vi "Destroy.vi"(0 "reference in":refnum<class "MessageAMC.lvclass">, 5 "error in (no error)":errorcluster) -> (14 "reference out":refnum<class "MessageAMC.lvclass">, 19 "error out":errorcluster)   [LabVIEW 2019, in "MessageAMC.lvclass"]
doc: "Destructor."
uses:
  MessageAMC.lvclass
  MessageAMC.lvclass/MessageAMC.ctl
  <vilib>/NI/AMC/AMC.lvlib
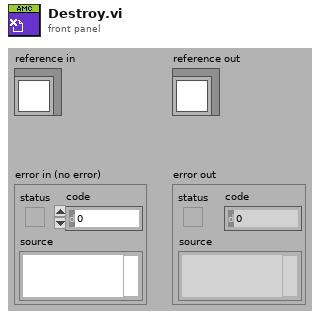
[diagram p1: front panel]
types:
  T1 = typedef "AMC.lvlib/Message Queue.ctl" = refnum<queue>
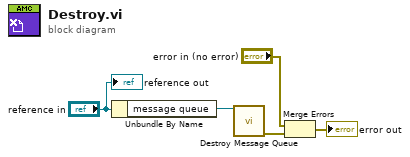
[diagram p0: block diagram]
diagram:
  n1 = Unbundle By Name("reference in") -> ("message queue"=w4:T1)
  n2 = call <vilib>:"Destroy Message Queue.vi"("message queue in"=w4) -> ("error out"=w3:errorcluster)  [unwired: 12 in, 2 out]
  n3 = Merge Errors("error in (no error)", w3) -> (→"error out":errorcluster)
  "reference out" <- "reference in"
